vi "READ BARCODE STRING FOR DATALOG.vi"(8 "error in (no error)":errorcluster, 11 "DECIMAL VALUE":u16[](array[numeric])) -> (0 "error out":errorcluster, 2 "String":string, 3 "ASCII VALUE":string[](array[string]))   [LabVIEW 2017]
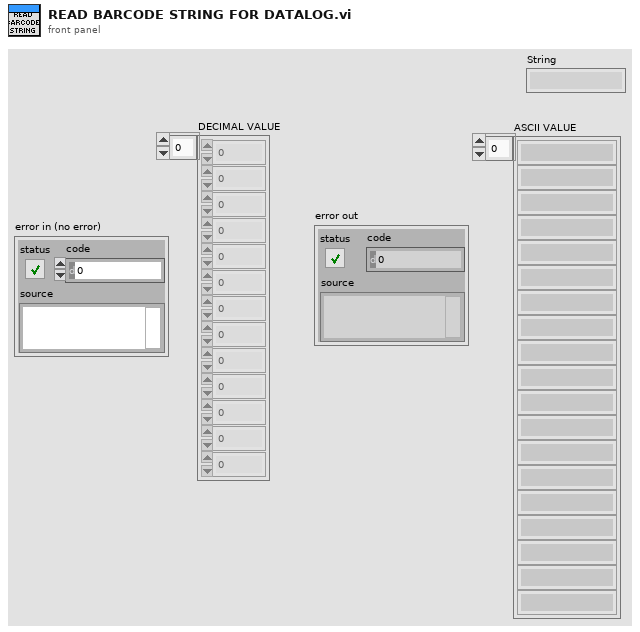
[diagram p1: front panel]
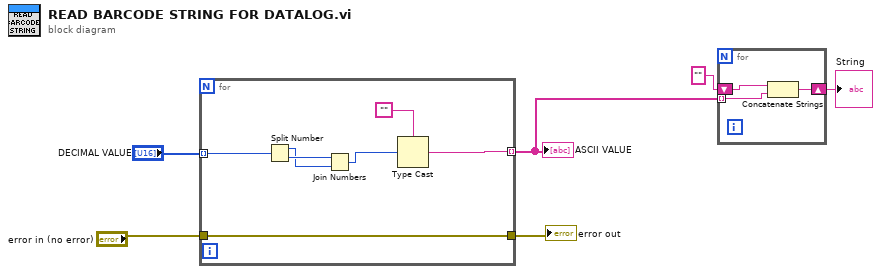
[diagram p0: block diagram]
diagram:
  n1 = for {
    tunnel: [w8] -> w2 mode=indexing
    tunnel: "DECIMAL VALUE" -> [w10] mode=indexing
    tunnel: [w7] -> w5
    tunnel: "error in (no error)" -> [w7]
    n2 = Split Number(x=w10) -> (hi(x)=w11:u8, lo(x)=w12:u8)
    n3 = Join Numbers(hi=w12, lo=w11) -> ((hi.lo)=w9:u16)
    n4 = Type Cast(type="", x=w9) -> (*(type *) &x=w8:string)
  }
  "ASCII VALUE" <- w2
  "error out" <- w5
  n5 = for {
    tunnel: w2 -> [w16] mode=indexing
    shift-right: [w15] -> w1
    shift-left: "" -> [w14]
    n6 = Concatenate Strings(w14, w16) -> (w15:string)
  }
  "String" <- w1
